vi "DAQ - Get Buffer Size (Samples).vi"(0 "reference in":refnum<class "GSwFormDSP.lvclass">, 5 "error in (no error)":errorcluster) -> (13 "Buffer Size (Samples)":i32, 14 "reference out":refnum<class "GSwFormDSP.lvclass">, 19 "error out":errorcluster)   [LabVIEW 2020, in "GSwFormDSP.lvclass"]
uses:
  GSwFormDSP.lvclass
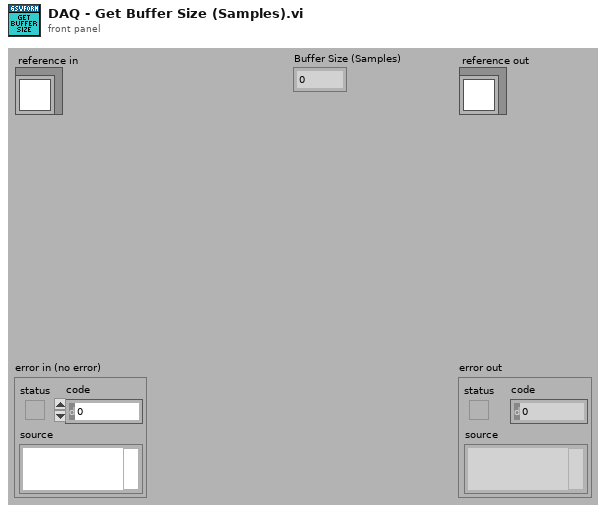
[diagram p1: front panel]
types:
  T1 = typedef "GSwFormDSP.lvclass/ObjectAttributes.ctl" = cluster{"Wform Ref":refnum<data-value>, "Nb Signals":i32, "Spectral Function Parameters":T2, "FFT":waveform(cdb)[], "Nb FFT":i32, "Nb Averages":i32[], "Reference Indexes":i32[], "Response Indexes":i32[], "Coherence":waveform(dbl)[], "TDF Parameters":T4, "DAQ":cluster{"Duration (sec)":dbl, "Buffer Size (Samples)":i32, "Offset (Samples)":i32}, "Filter Impulse Response (TDF)":waveform(dbl), "Sound Playback":T5}
  T2 = typedef "GSwFormDSP.lvclass/Spectral Parameters.ctl" = cluster{"Frequency resolution (Hz)":dbl, "Overlap":dbl, "Window":T3}
  T3 = typedef "NI_AALPro.lvlib/windowTd.ctl" = u32
  T4 = typedef "GSwFormDSP.lvclass/TDF Parameters.ctl" = cluster{"Filter":enum32{"Lowpass", "Highpass", "Bandpass", "Bandstop"}, "Type:":enum16{"Butterworth", "Chebyshev", "Inv Chebyshev", "Elliptic", "Bessel"}, "LP cutoff freq":dbl, "HP cutoff freq":dbl, "Order":i32, "passband ripple (dB)":dbl, "stopband attenuation (dB)":dbl, "Phaseless Filter":bool, "Include Fade IN and OUT":bool}
  T5 = typedef "GSwFormDSP.lvclass/Sound Playback.ctl" = cluster{"Timer start (ms)":u32, "task ID":T6, "Cursor Init Location (s)":dbl, "SC Volume":dbl}
  T6 = typedef "Sound Output Task ID.ctl" = u32
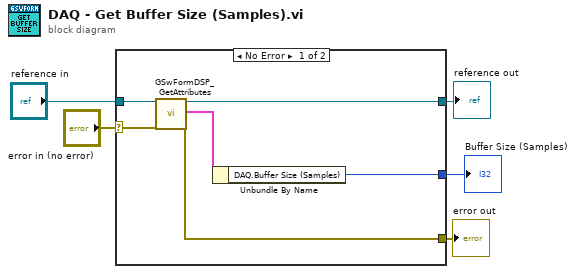
[diagram p0: block diagram]
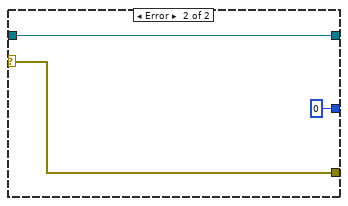
[diagram p2: hidden frame]
diagram:
  n1 = case shown="No Error" "error in (no error)" {
    selector: "error in (no error)" -> [w11 w14]
    tunnel: [w10 w14] -> w4
    tunnel: [w9 w13] -> w2
    tunnel: "reference in" -> [w7 w13]
    tunnel: [w6 0 ("Duration (sec)")] -> w1
    frame No Error {
      n2 = call "GSwFormDSP_GetAttributes.vi"("reference in"=w7, "error in (no error)"=w11) -> ("reference out"=w9:refnum<class "GSwFormDSP.lvclass">, "attributes"=w8:T1, "error out"=w10:errorcluster)  [unwired: 14 in, 1 out]
      n3 = Unbundle By Name(w8) -> ("DAQ.Buffer Size (Samples)"=w6:i32)
    }
    frame Error {
    }
  }
  "error out" <- w4
  "reference out" <- w2
  "Buffer Size (Samples)" <- w1
